vi "GA Cmp Rpt.vi"(4 "nTime":i16, 5 "lInterval":i32, 6 "lRptTime":i32, 7 "lStartPos":i32, 8 "error in (no error)":errorcluster caption="错误输入（无错误）", 9 "nChannel":i16, 10 "nEncodeType":i16, 11 "nEncode":i16) -> (0 "error out":errorcluster caption="错误输出", 3 "function return":i32)   [LabVIEW 2015, in "GAS.lvlib"]
doc: "extern \"C\" __declspec(dllimport) int GA_CmpRpt(short nEncode, short nEncodeType,short nChannel,long lStartPos, long lRptTime, long lInterval, short nTime);"
uses:
  <userlib>/BP_GAS/GAS.lvlib
  <userlib>/BP_GAS/GAS.dll
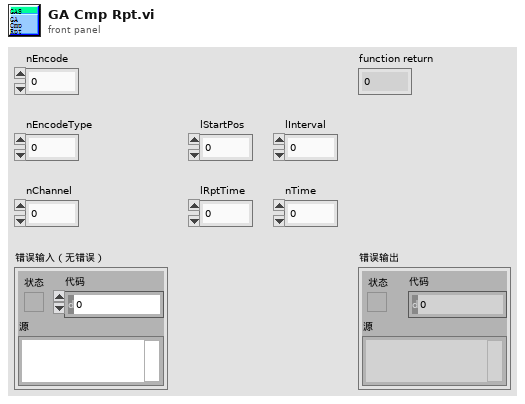
[diagram p1: front panel]
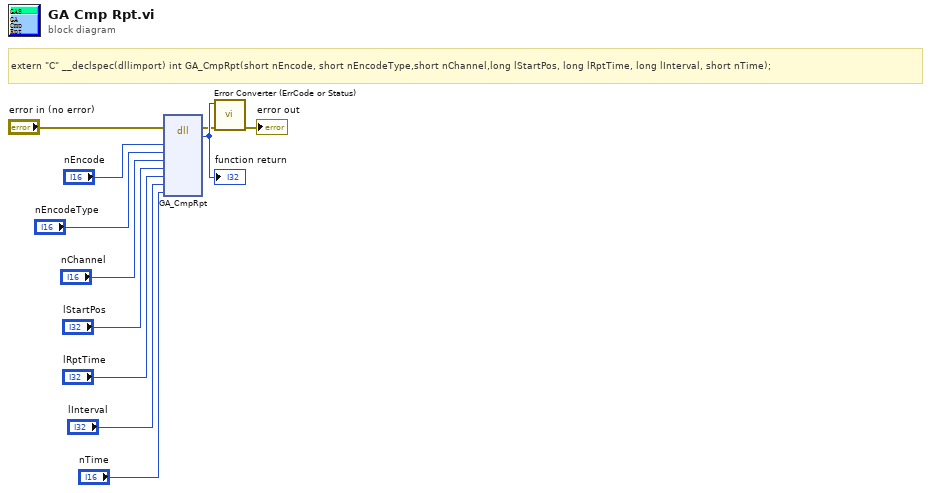
[diagram p0: block diagram]
diagram:
  # "extern \"C\" __declspec(dllimport) int GA_CmpRpt(short nEncode, short nEncodeType,short nChannel,long lStartPos, long lRptTime, long lInterval, short nTime);"
  n1 = dll-call lib="E:/Program Files (x86)/National Instruments/LabVIEW 2015/user.lib/BP_GAS/GAS.*" fn="GA_CmpRpt"(error in="error in (no error)", "nEncode"="nEncode", "nEncodeType"="nEncodeType", "nChannel"="nChannel", "lStartPos"="lStartPos", "lRptTime"="lRptTime", "lInterval"="lInterval", "nTime"="nTime") -> (error out=w2:errorcluster, w11:i32)  [unwired: 9 in, 1 out]
  "function return" <- w11
  n2 = call "Error Converter (ErrCode or Status).vi"("error in (no error)"=w2, "error code"=w11) -> ("error out"=→"error out":errorcluster)  [unwired: 9 in]
